vi "FeedbackDecode.vi"() -> ()   [LabVIEW 2020] (continued)
            n2136 = call "FeedbackDecode_MLComCtrl.vi"("DecodeClustIn"=w2282, "Mode"=T19."SendEvent") -> ()  [unwired: 6 in, 4 out]
          }
          event Value Change {
            n2137 = event-data() -> ()  [unwired: 1 in, 6 out]
            n2138 = local read "EncodeClust"() -> (w2298:T9)
            n2139 = call "FeedbackDecode_AdjParamsTable.vi"("StimClustIn"=w2298, "Mode"=enum16{"Set", "Add", "Sub"}."Add") -> ("StimClustOut"=w2296:T9)  [unwired: 1 in]
            n2140 = Bundle By Name(cluster=w2296, "AdjClust.Add"=FALSE ("AdjClust.Set")) -> (w2294:T9)
            n2141 = local read "LoopCnt"() -> (w2308:u64)
            n2142 = call "FeedbackDecode_Params2Preset.vi"("StimClustIn"=w2294) -> ("StimClustOut"=w2299:T9)  [unwired: 2 in]
            n2143 = Format Into String(w2308) -> (resulting string=w2300:string)  [unwired: 3 in, 1 out]
            n2144 = local read "NIPTime"() -> (w2304:dbl)
            n2145 = call "FeedbackDecode_BuildStimCmd.vi"("EncodeClustIn"=w2299) -> ("EncodeClustOut"=w2314:T9, "StimCmd"=w2293:string)  [unwired: 1 in]
            n2146 = local read "EventParamsFID"() -> (w2312:refnum<file>)
            n2147 = Concatenate Strings("UpdateStim:SS.EventID=" ("string"), w2300) -> (w2307:string)
            n2148 = call-poly "FeedbackDecode_VariablesToString.vi"("Format"="%0.0f", "ValueIn"=w2304, "FieldName"="NIPTime" ("Key Word")) -> ("StringOut"=w2301:string)  [unwired: 4 in]
            n2149 = local read "DecodeClust"() -> (w2313:T5)
            n2150 = Concatenate Strings(w2307, ";", w2293, w2301) -> (w2306:string)
            n2151 = call "FeedbackDecode_WriteTextEOL.vi"("text"=w2306, "refnum in"=w2312) -> ()  [unwired: 8 in, 2 out]
            n2152 = Bundle By Name(cluster=w2313, "EventStr"=w2306) -> (w2305:T5)
            n2153 = local write "StimCmd"(w2293) -> ()
            n2154 = local write "EncodeClust"(w2314) -> ()
            n2155 = call "FeedbackDecode_MLComCtrl.vi"("DecodeClustIn"=w2305, "Mode"=T19."SendEvent") -> ()  [unwired: 6 in, 4 out]
          }
          event Value Change {
            n2156 = event-data() -> ()  [unwired: 1 in, 6 out]
            n2157 = local read "EncodeClust"() -> (w2321:T9)
            n2158 = call "FeedbackDecode_AdjParamsTable.vi"("StimClustIn"=w2321, "Mode"=enum16{"Set", "Add", "Sub"}."Sub") -> ("StimClustOut"=w2319:T9)  [unwired: 1 in]
            n2159 = Bundle By Name(cluster=w2319, "AdjClust.Sub"=FALSE ("AdjClust.Set")) -> (w2317:T9)
            n2160 = local read "LoopCnt"() -> (w2331:u64)
            n2161 = call "FeedbackDecode_Params2Preset.vi"("StimClustIn"=w2317) -> ("StimClustOut"=w2322:T9)  [unwired: 2 in]
            n2162 = Format Into String(w2331) -> (resulting string=w2323:string)  [unwired: 3 in, 1 out]
            n2163 = local read "NIPTime"() -> (w2327:dbl)
            n2164 = call "FeedbackDecode_BuildStimCmd.vi"("EncodeClustIn"=w2322) -> ("EncodeClustOut"=w2337:T9, "StimCmd"=w2316:string)  [unwired: 1 in]
            n2165 = local read "EventParamsFID"() -> (w2335:refnum<file>)
            n2166 = Concatenate Strings("UpdateStim:SS.EventID=" ("string"), w2323) -> (w2330:string)
            n2167 = call-poly "FeedbackDecode_VariablesToString.vi"("Format"="%0.0f", "ValueIn"=w2327, "FieldName"="NIPTime" ("Key Word")) -> ("StringOut"=w2324:string)  [unwired: 4 in]
            n2168 = local read "DecodeClust"() -> (w2336:T5)
            n2169 = Concatenate Strings(w2330, ";", w2316, w2324) -> (w2329:string)
            n2170 = call "FeedbackDecode_WriteTextEOL.vi"("text"=w2329, "refnum in"=w2335) -> ()  [unwired: 8 in, 2 out]
            n2171 = Bundle By Name(cluster=w2336, "EventStr"=w2329) -> (w2328:T5)
            n2172 = local write "StimCmd"(w2316) -> ()
            n2173 = local write "EncodeClust"(w2337) -> ()
            n2174 = call "FeedbackDecode_MLComCtrl.vi"("DecodeClustIn"=w2328, "Mode"=T19."SendEvent") -> ()  [unwired: 6 in, 4 out]
          }
          event Value Change {
            n2175 = event-data() -> ()  [unwired: 1 in, 6 out]
            n2176 = local read "EncodeClust"() -> (w2351:T9)
            n2177 = Unbundle By Name(w2351) -> ("Sel"=w2344:bool[], "ParamsTable"=w2345:string[][], "SelPreset"=w2349:bool[])
            n2178 = while {
              shift-right: [w2377] -> w2343
              shift-left: w2344 -> [w2376]
              shift-right: [w2372] -> w2342
              shift-left: w2345 -> [w2373]
              stop <- w2370 stop-if-true
              n2179 = Search 1D Array(1D array=w2376, element=TRUE) -> (index of element=w2371:i32)  [unwired: 1 in]
              n2180 = Less Than 0?(x=w2371) -> (x < 0?=w2370:bool)
              n2181 = Delete From Array(array=w2376, length=1, index=w2371) -> (array with subset deleted=w2377:bool[])  [unwired: 1 out]
              n2182 = Delete From Array(array=w2373, length=1, index (row)=w2371) -> (array with subset deleted=w2372:string[][])  [unwired: 1 in, 1 out]
            }
            n2183 = Array Size(array=w2349) -> (size(s)=w2347:i32)
            n2184 = Initialize Array(FALSE, w2347) -> (w2350:bool[])
            n2185 = Bundle By Name(cluster=w2351, "Sel"=w2343, "ParamsTable"=w2342, "AdjClust.DeleteSel"=FALSE, "SelPreset"=w2350) -> (w2341:T9)
            n2186 = local read "LoopCnt"() -> (w2361:u64)
            n2187 = call "FeedbackDecode_UpdateParamsTable.vi"("StimClustIn"=w2341) -> ("StimClustOut"=w2340:T9)  [unwired: 2 in]
            n2188 = call "FeedbackDecode_Params2UEA.vi"("StimClustIn"=w2340) -> ("StimClustOut"=w2352:T9)  [unwired: 2 in]
            n2189 = Format Into String(w2361) -> (resulting string=w2353:string)  [unwired: 3 in, 1 out]
            n2190 = local read "NIPTime"() -> (w2357:dbl)
            n2191 = call "FeedbackDecode_BuildStimCmd.vi"("EncodeClustIn"=w2352) -> ("EncodeClustOut"=w2367:T9, "StimCmd"=w2339:string)  [unwired: 1 in]
            n2192 = local read "EventParamsFID"() -> (w2365:refnum<file>)
            n2193 = Concatenate Strings("DelStimParam:SS.EventID=" ("string"), w2353) -> (w2360:string)
            n2194 = call-poly "FeedbackDecode_VariablesToString.vi"("Format"="%0.0f", "ValueIn"=w2357, "FieldName"="NIPTime" ("Key Word")) -> ("StringOut"=w2354:string)  [unwired: 4 in]
            n2195 = local read "DecodeClust"() -> (w2366:T5)
            n2196 = Concatenate Strings(w2360, ";", w2339, w2354) -> (w2359:string)
            n2197 = call "FeedbackDecode_WriteTextEOL.vi"("text"=w2359, "refnum in"=w2365) -> ()  [unwired: 8 in, 2 out]
            n2198 = Bundle By Name(cluster=w2366, "EventStr"=w2359) -> (w2358:T5)
            n2199 = local write "StimCmd"(w2339) -> ()
            n2200 = local write "EncodeClust"(w2367) -> ()
            n2201 = call "FeedbackDecode_MLComCtrl.vi"("DecodeClustIn"=w2358, "Mode"=T19."SendEvent") -> ()  [unwired: 6 in, 4 out]
          }
          event Value Change {
            n2202 = event-data() -> ()  [unwired: 1 in, 6 out]
            n2203 = local read "EncodeClust"() -> (w2391:T9)
            n2204 = Unbundle By Name(w2391) -> ("SelPreset"=w2384:bool[], "PresetTable"=w2385:string[][], "Sel"=w2389:bool[])
            n2205 = while {
              shift-right: [w2417] -> w2383
              shift-left: w2384 -> [w2416]
              shift-right: [w2412] -> w2382
              shift-left: w2385 -> [w2413]
              stop <- w2410 stop-if-true
              n2206 = Search 1D Array(1D array=w2416, element=TRUE) -> (index of element=w2411:i32)  [unwired: 1 in]
              n2207 = Less Than 0?(x=w2411) -> (x < 0?=w2410:bool)
              n2208 = Delete From Array(array=w2416, length=1, index=w2411) -> (array with subset deleted=w2417:bool[])  [unwired: 1 out]
              n2209 = Delete From Array(array=w2413, length=1, index (row)=w2411) -> (array with subset deleted=w2412:string[][])  [unwired: 1 in, 1 out]
            }
            n2210 = Array Size(array=w2389) -> (size(s)=w2387:i32)
            n2211 = Initialize Array(FALSE, w2387) -> (w2390:bool[])
            n2212 = Bundle By Name(cluster=w2391, "SelPreset"=w2383, "PresetTable"=w2382, "PresetClust.Del"=FALSE ("AdjClust.DeleteSel"), "Sel"=w2390) -> (w2379:T9)
            n2213 = call "FeedbackDecode_UpdatePresetsTable.vi"("StimClustIn"=w2379) -> ("StimClustOut"=w2378:T9)  [unwired: 2 in]
            n2214 = local read "LoopCnt"() -> (w2401:u64)
            n2215 = call "FeedbackDecode_UpdateParamsTable.vi"("StimClustIn"=w2378) -> ("StimClustOut"=w2381:T9)  [unwired: 2 in]
            n2216 = call "FeedbackDecode_Params2UEA.vi"("StimClustIn"=w2381) -> ("StimClustOut"=w2392:T9)  [unwired: 2 in]
            n2217 = Format Into String(w2401) -> (resulting string=w2393:string)  [unwired: 3 in, 1 out]
            n2218 = local read "NIPTime"() -> (w2397:dbl)
            n2219 = call "FeedbackDecode_BuildStimCmd.vi"("EncodeClustIn"=w2392) -> ("EncodeClustOut"=w2407:T9, "StimCmd"=w2380:string)  [unwired: 1 in]
            n2220 = local read "EventParamsFID"() -> (w2405:refnum<file>)
            n2221 = Concatenate Strings("DelPreset:SS.EventID=" ("string"), w2393) -> (w2400:string)
            n2222 = call-poly "FeedbackDecode_VariablesToString.vi"("Format"="%0.0f", "ValueIn"=w2397, "FieldName"="NIPTime" ("Key Word")) -> ("StringOut"=w2394:string)  [unwired: 4 in]
            n2223 = local read "DecodeClust"() -> (w2406:T5)
            n2224 = Concatenate Strings(w2400, ";", w2380, w2394) -> (w2399:string)
            n2225 = call "FeedbackDecode_WriteTextEOL.vi"("text"=w2399, "refnum in"=w2405) -> ()  [unwired: 8 in, 2 out]
            n2226 = Bundle By Name(cluster=w2406, "EventStr"=w2399) -> (w2398:T5)
            n2227 = local write "StimCmd"(w2380) -> ()
            n2228 = local write "EncodeClust"(w2407) -> ()
            n2229 = call "FeedbackDecode_MLComCtrl.vi"("DecodeClustIn"=w2398, "Mode"=T19."SendEvent") -> ()  [unwired: 6 in, 4 out]
          }
          event Value Change {
            n2230 = event-data() -> ()  [unwired: 1 in, 6 out]
            n2231 = local read "EncodeClust"() -> (w2428:T9)
            n2232 = Unbundle By Name(w2428) -> ("SelPreset"=w2424:bool[])
            n2233 = Array Size(array=w2424) -> (size(s)=w2426:i32)
            n2234 = Initialize Array(FALSE, w2426) -> (w2427:bool[])
            n2235 = Bundle By Name(cluster=w2428, "ParamsTable"=string[][] [], "Sel"=bool[] [], "UEAArray"=T25 [{"Boolean 1"=FALSE, "Boolean 2"=FALSE, "Boolean 3"=FALSE, "Boolean 4"=FALSE, "Boolean 5"=FALSE, "Boolean 6"=FALSE, "Boolean 7"=FALSE, "Boolean 8"=FALSE, "Boolean 9"=FALSE, "Boolean 10"=FALSE, "Boolean 11"=FALSE, "Boolean 12"=FALSE, "Boolean 13"=FALSE, "Boolean 14"=FALSE, "Boolean 15"=FALSE, "Boolean 16"=FALSE, "Boolean 17"=FALSE, "Boolean 18"=FALSE, "Boolean 19"=FALSE, "Boolean 20"=FALSE, "Boolean 21"=FALSE, "Boolean 22"=FALSE, "Boolean 23"=FALSE, "Boolean 24"=FALSE, "Boolean 25"=FALSE, "Boolean 26"=FALSE, "Boolean 27"=FALSE, "Boolean 28"=FALSE, "Boolean 29"=FALSE, "Boolean 30"=FALSE, "Boolean 31"=FALSE, "Boolean 32"=FALSE, "Boolean 33"=FALSE, "Boolean 34"=FALSE, "Boolean 35"=FALSE, "Boolean 36"=FALSE, "Boolean 37"=FALSE, "Boolean 38"=FALSE, "Boolean 39"=FALSE, "Boolean 40"=FALSE, "Boolean 41"=FALSE, "Boolean 42"=FALSE, "Boolean 43"=FALSE, "Boolean 44"=FALSE, "Boolean 45"=FALSE, "Boolean 46"=FALSE, "Boolean 47"=FALSE, "Boolean 48"=FALSE, "Boolean 49"=FALSE, "Boolean 50"=FALSE, "Boolean 51"=FALSE, "Boolean 52"=FALSE, "Boolean 53"=FALSE, "Boolean 54"=FALSE, "Boolean 55"=FALSE, "Boolean 56"=FALSE, "Boolean 57"=FALSE, "Boolean 58"=FALSE, "Boolean 59"=FALSE, "Boolean 60"=FALSE, "Boolean 61"=FALSE, "Boolean 62"=FALSE, "Boolean 63"=FALSE, "Boolean 64"=FALSE, "Boolean 65"=FALSE, "Boolean 66"=FALSE, "Boolean 67"=FALSE, "Boolean 68"=FALSE, "Boolean 69"=FALSE, "Boolean 70"=FALSE, "Boolean 71"=FALSE, "Boolean 72"=FALSE, "Boolean 73"=FALSE, "Boolean 74"=FALSE, "Boolean 75"=FALSE, "Boolean 76"=FALSE, "Boolean 77"=FALSE, "Boolean 78"=FALSE, "Boolean 79"=FALSE, "Boolean 80"=FALSE, "Boolean 81"=FALSE, "Boolean 82"=FALSE, "Boolean 83"=FALSE, "Boolean 84"=FALSE, "Boolean 85"=FALSE, "Boolean 86"=FALSE, "Boolean 87"=FALSE, "Boolean 88"=FALSE, "Boolean 89"=FALSE, "Boolean 90"=FALSE, "Boolean 91"=FALSE, "Boolean 92"=FALSE, "Boolean 93"=FALSE, "Boolean 94"=FALSE, "Boolean 95"=FALSE, "Boolean 96"=FALSE, "Boolean 97"=FALSE, "Boolean 98"=FALSE, "Boolean 99"=FALSE, "Boolean 100"=FALSE}, {"Boolean 1"=FALSE, "Boolean 2"=FALSE, "Boolean 3"=FALSE, "Boolean 4"=FALSE, "Boolean 5"=FALSE, "Boolean 6"=FALSE, "Boolean 7"=FALSE, "Boolean 8"=FALSE, "Boolean 9"=FALSE, "Boolean 10"=FALSE, "Boolean 11"=FALSE, "Boolean 12"=FALSE, "Boolean 13"=FALSE, "Boolean 14"=FALSE, "Boolean 15"=FALSE, "Boolean 16"=FALSE, "Boolean 17"=FALSE, "Boolean 18"=FALSE, "Boolean 19"=FALSE, "Boolean 20"=FALSE, "Boolean 21"=FALSE, "Boolean 22"=FALSE, "Boolean 23"=FALSE, "Boolean 24"=FALSE, "Boolean 25"=FALSE, "Boolean 26"=FALSE, "Boolean 27"=FALSE, "Boolean 28"=FALSE, "Boolean 29"=FALSE, "Boolean 30"=FALSE, "Boolean 31"=FALSE, "Boolean 32"=FALSE, "Boolean 33"=FALSE, "Boolean 34"=FALSE, "Boolean 35"=FALSE, "Boolean 36"=FALSE, "Boolean 37"=FALSE, "Boolean 38"=FALSE, "Boolean 39"=FALSE, "Boolean 40"=FALSE, "Boolean 41"=FALSE, "Boolean 42"=FALSE, "Boolean 43"=FALSE, "Boolean 44"=FALSE, "Boolean 45"=FALSE, "Boolean 46"=FALSE, "Boolean 47"=FALSE, "Boolean 48"=FALSE, "Boolean 49"=FALSE, "Boolean 50"=FALSE, "Boolean 51"=FALSE, "Boolean 52"=FALSE, "Boolean 53"=FALSE, "Boolean 54"=FALSE, "Boolean 55"=FALSE, "Boolean 56"=FALSE, "Boolean 57"=FALSE, "Boolean 58"=FALSE, "Boolean 59"=FALSE, "Boolean 60"=FALSE, "Boolean 61"=FALSE, "Boolean 62"=FALSE, "Boolean 63"=FALSE, "Boolean 64"=FALSE, "Boolean 65"=FALSE, "Boolean 66"=FALSE, "Boolean 67"=FALSE, "Boolean 68"=FALSE, "Boolean 69"=FALSE, "Boolean 70"=FALSE, "Boolean 71"=FALSE, "Boolean 72"=FALSE, "Boolean 73"=FALSE, "Boolean 74"=FALSE, "Boolean 75"=FALSE, "Boolean 76"=FALSE, "Boolean 77"=FALSE, "Boolean 78"=FALSE, "Boolean 79"=FALSE, "Boolean 80"=FALSE, "Boolean 81"=FALSE, "Boolean 82"=FALSE, "Boolean 83"=FALSE, "Boolean 84"=FALSE, "Boolean 85"=FALSE, "Boolean 86"=FALSE, "Boolean 87"=FALSE, "Boolean 88"=FALSE, "Boolean 89"=FALSE, "Boolean 90"=FALSE, "Boolean 91"=FALSE, "Boolean 92"=FALSE, "Boolean 93"=FALSE, "Boolean 94"=FALSE, "Boolean 95"=FALSE, "Boolean 96"=FALSE, "Boolean 97"=FALSE, "Boolean 98"=FALSE, "Boolean 99"=FALSE, "Boolean 100"=FALSE}], "AdjClust.ClearTable"=FALSE, "SelPreset"=w2427) -> (w2419:T9)
            n2236 = local read "LoopCnt"() -> (w2439:u64)
            n2237 = call "FeedbackDecode_UpdateParamsTable.vi"("StimClustIn"=w2419) -> ("StimClustOut"=w2429:T9)  [unwired: 2 in]
            n2238 = call "FeedbackDecode_Params2UEA.vi"("StimClustIn"=w2429) -> ("StimClustOut"=w2430:T9)  [unwired: 2 in]
            n2239 = Format Into String(w2439) -> (resulting string=w2431:string)  [unwired: 3 in, 1 out]
            n2240 = local read "NIPTime"() -> (w2435:dbl)
            n2241 = call "FeedbackDecode_BuildStimCmd.vi"("EncodeClustIn"=w2430) -> ("EncodeClustOut"=w2445:T9, "StimCmd"=w2418:string)  [unwired: 1 in]
            n2242 = local read "EventParamsFID"() -> (w2443:refnum<file>)
            n2243 = Concatenate Strings("ClearStimParams:SS.EventID=" ("string"), w2431) -> (w2438:string)
            n2244 = call-poly "FeedbackDecode_VariablesToString.vi"("Format"="%0.0f", "ValueIn"=w2435, "FieldName"="NIPTime" ("Key Word")) -> ("StringOut"=w2432:string)  [unwired: 4 in]
            n2245 = local read "DecodeClust"() -> (w2444:T5)
            n2246 = Concatenate Strings(w2438, ";", w2418, w2432) -> (w2437:string)
            n2247 = call "FeedbackDecode_WriteTextEOL.vi"("text"=w2437, "refnum in"=w2443) -> ()  [unwired: 8 in, 2 out]
            n2248 = Bundle By Name(cluster=w2444, "EventStr"=w2437) -> (w2436:T5)
            n2249 = local write "StimCmd"(w2418) -> ()
            n2250 = local write "EncodeClust"(w2445) -> ()
            n2251 = call "FeedbackDecode_MLComCtrl.vi"("DecodeClustIn"=w2436, "Mode"=T19."SendEvent") -> ()  [unwired: 6 in, 4 out]
          }
          event Value Change {
            n2252 = event-data() -> ()  [unwired: 1 in, 6 out]
            n2253 = local read "EncodeClust"() -> (w2458:T9)
            n2254 = Unbundle By Name(w2458) -> ("Sel"=w2454:bool[])
            n2255 = Array Size(array=w2454) -> (size(s)=w2456:i32)
            n2256 = Initialize Array(FALSE, w2456) -> (w2457:bool[])
            n2257 = Bundle By Name(cluster=w2458, "PresetTable"=string[][] [] ("ParamsTable"), "SelPreset"=bool[] [] ("Sel"), "UEAArray"=T25 [{"Boolean 1"=FALSE, "Boolean 2"=FALSE, "Boolean 3"=FALSE, "Boolean 4"=FALSE, "Boolean 5"=FALSE, "Boolean 6"=FALSE, "Boolean 7"=FALSE, "Boolean 8"=FALSE, "Boolean 9"=FALSE, "Boolean 10"=FALSE, "Boolean 11"=FALSE, "Boolean 12"=FALSE, "Boolean 13"=FALSE, "Boolean 14"=FALSE, "Boolean 15"=FALSE, "Boolean 16"=FALSE, "Boolean 17"=FALSE, "Boolean 18"=FALSE, "Boolean 19"=FALSE, "Boolean 20"=FALSE, "Boolean 21"=FALSE, "Boolean 22"=FALSE, "Boolean 23"=FALSE, "Boolean 24"=FALSE, "Boolean 25"=FALSE, "Boolean 26"=FALSE, "Boolean 27"=FALSE, "Boolean 28"=FALSE, "Boolean 29"=FALSE, "Boolean 30"=FALSE, "Boolean 31"=FALSE, "Boolean 32"=FALSE, "Boolean 33"=FALSE, "Boolean 34"=FALSE, "Boolean 35"=FALSE, "Boolean 36"=FALSE, "Boolean 37"=FALSE, "Boolean 38"=FALSE, "Boolean 39"=FALSE, "Boolean 40"=FALSE, "Boolean 41"=FALSE, "Boolean 42"=FALSE, "Boolean 43"=FALSE, "Boolean 44"=FALSE, "Boolean 45"=FALSE, "Boolean 46"=FALSE, "Boolean 47"=FALSE, "Boolean 48"=FALSE, "Boolean 49"=FALSE, "Boolean 50"=FALSE, "Boolean 51"=FALSE, "Boolean 52"=FALSE, "Boolean 53"=FALSE, "Boolean 54"=FALSE, "Boolean 55"=FALSE, "Boolean 56"=FALSE, "Boolean 57"=FALSE, "Boolean 58"=FALSE, "Boolean 59"=FALSE, "Boolean 60"=FALSE, "Boolean 61"=FALSE, "Boolean 62"=FALSE, "Boolean 63"=FALSE, "Boolean 64"=FALSE, "Boolean 65"=FALSE, "Boolean 66"=FALSE, "Boolean 67"=FALSE, "Boolean 68"=FALSE, "Boolean 69"=FALSE, "Boolean 70"=FALSE, "Boolean 71"=FALSE, "Boolean 72"=FALSE, "Boolean 73"=FALSE, "Boolean 74"=FALSE, "Boolean 75"=FALSE, "Boolean 76"=FALSE, "Boolean 77"=FALSE, "Boolean 78"=FALSE, "Boolean 79"=FALSE, "Boolean 80"=FALSE, "Boolean 81"=FALSE, "Boolean 82"=FALSE, "Boolean 83"=FALSE, "Boolean 84"=FALSE, "Boolean 85"=FALSE, "Boolean 86"=FALSE, "Boolean 87"=FALSE, "Boolean 88"=FALSE, "Boolean 89"=FALSE, "Boolean 90"=FALSE, "Boolean 91"=FALSE, "Boolean 92"=FALSE, "Boolean 93"=FALSE, "Boolean 94"=FALSE, "Boolean 95"=FALSE, "Boolean 96"=FALSE, "Boolean 97"=FALSE, "Boolean 98"=FALSE, "Boolean 99"=FALSE, "Boolean 100"=FALSE}, {"Boolean 1"=FALSE, "Boolean 2"=FALSE, "Boolean 3"=FALSE, "Boolean 4"=FALSE, "Boolean 5"=FALSE, "Boolean 6"=FALSE, "Boolean 7"=FALSE, "Boolean 8"=FALSE, "Boolean 9"=FALSE, "Boolean 10"=FALSE, "Boolean 11"=FALSE, "Boolean 12"=FALSE, "Boolean 13"=FALSE, "Boolean 14"=FALSE, "Boolean 15"=FALSE, "Boolean 16"=FALSE, "Boolean 17"=FALSE, "Boolean 18"=FALSE, "Boolean 19"=FALSE, "Boolean 20"=FALSE, "Boolean 21"=FALSE, "Boolean 22"=FALSE, "Boolean 23"=FALSE, "Boolean 24"=FALSE, "Boolean 25"=FALSE, "Boolean 26"=FALSE, "Boolean 27"=FALSE, "Boolean 28"=FALSE, "Boolean 29"=FALSE, "Boolean 30"=FALSE, "Boolean 31"=FALSE, "Boolean 32"=FALSE, "Boolean 33"=FALSE, "Boolean 34"=FALSE, "Boolean 35"=FALSE, "Boolean 36"=FALSE, "Boolean 37"=FALSE, "Boolean 38"=FALSE, "Boolean 39"=FALSE, "Boolean 40"=FALSE, "Boolean 41"=FALSE, "Boolean 42"=FALSE, "Boolean 43"=FALSE, "Boolean 44"=FALSE, "Boolean 45"=FALSE, "Boolean 46"=FALSE, "Boolean 47"=FALSE, "Boolean 48"=FALSE, "Boolean 49"=FALSE, "Boolean 50"=FALSE, "Boolean 51"=FALSE, "Boolean 52"=FALSE, "Boolean 53"=FALSE, "Boolean 54"=FALSE, "Boolean 55"=FALSE, "Boolean 56"=FALSE, "Boolean 57"=FALSE, "Boolean 58"=FALSE, "Boolean 59"=FALSE, "Boolean 60"=FALSE, "Boolean 61"=FALSE, "Boolean 62"=FALSE, "Boolean 63"=FALSE, "Boolean 64"=FALSE, "Boolean 65"=FALSE, "Boolean 66"=FALSE, "Boolean 67"=FALSE, "Boolean 68"=FALSE, "Boolean 69"=FALSE, "Boolean 70"=FALSE, "Boolean 71"=FALSE, "Boolean 72"=FALSE, "Boolean 73"=FALSE, "Boolean 74"=FALSE, "Boolean 75"=FALSE, "Boolean 76"=FALSE, "Boolean 77"=FALSE, "Boolean 78"=FALSE, "Boolean 79"=FALSE, "Boolean 80"=FALSE, "Boolean 81"=FALSE, "Boolean 82"=FALSE, "Boolean 83"=FALSE, "Boolean 84"=FALSE, "Boolean 85"=FALSE, "Boolean 86"=FALSE, "Boolean 87"=FALSE, "Boolean 88"=FALSE, "Boolean 89"=FALSE, "Boolean 90"=FALSE, "Boolean 91"=FALSE, "Boolean 92"=FALSE, "Boolean 93"=FALSE, "Boolean 94"=FALSE, "Boolean 95"=FALSE, "Boolean 96"=FALSE, "Boolean 97"=FALSE, "Boolean 98"=FALSE, "Boolean 99"=FALSE, "Boolean 100"=FALSE}], "PresetClust.Clear"=FALSE ("AdjClust.ClearTable"), "Sel"=w2457) -> (w2448:T9)
            n2258 = call "FeedbackDecode_UpdatePresetsTable.vi"("StimClustIn"=w2448) -> ("StimClustOut"=w2447:T9)  [unwired: 2 in]
            n2259 = local read "LoopCnt"() -> (w2469:u64)
            n2260 = call "FeedbackDecode_UpdateParamsTable.vi"("StimClustIn"=w2447) -> ("StimClustOut"=w2459:T9)  [unwired: 2 in]
            n2261 = call "FeedbackDecode_Params2UEA.vi"("StimClustIn"=w2459) -> ("StimClustOut"=w2460:T9)  [unwired: 2 in]
            n2262 = Format Into String(w2469) -> (resulting string=w2461:string)  [unwired: 3 in, 1 out]
            n2263 = local read "NIPTime"() -> (w2465:dbl)
            n2264 = call "FeedbackDecode_BuildStimCmd.vi"("EncodeClustIn"=w2460) -> ("EncodeClustOut"=w2475:T9, "StimCmd"=w2449:string)  [unwired: 1 in]
            n2265 = local read "EventParamsFID"() -> (w2473:refnum<file>)
            n2266 = Concatenate Strings("ClearPresets:SS.EventID=" ("string"), w2461) -> (w2468:string)
            n2267 = call-poly "FeedbackDecode_VariablesToString.vi"("Format"="%0.0f", "ValueIn"=w2465, "FieldName"="NIPTime" ("Key Word")) -> ("StringOut"=w2462:string)  [unwired: 4 in]
            n2268 = local read "DecodeClust"() -> (w2474:T5)
            n2269 = Concatenate Strings(w2468, ";", w2449, w2462) -> (w2467:string)
            n2270 = call "FeedbackDecode_WriteTextEOL.vi"("text"=w2467, "refnum in"=w2473) -> ()  [unwired: 8 in, 2 out]
            n2271 = Bundle By Name(cluster=w2474, "EventStr"=w2467) -> (w2466:T5)
            n2272 = local write "StimCmd"(w2449) -> ()
            n2273 = local write "EncodeClust"(w2475) -> ()
            n2274 = call "FeedbackDecode_MLComCtrl.vi"("DecodeClustIn"=w2466, "Mode"=T19."SendEvent") -> ()  [unwired: 6 in, 4 out]
          }
          event Value Change {
            n2275 = event-data() -> ()  [unwired: 1 in, 6 out]
            n2276 = local read "EncodeClust"() -> (w2485:T9)
            n2277 = Bundle By Name(cluster=w2485, "Stim"=FALSE) -> (w2483:T9)
            n2278 = call "FeedbackDecode_BuildStimCmd.vi"("EncodeClustIn"=w2483) -> ("EncodeClustOut"=w2495:T9, "StimCmd"=w2477:string)  [unwired: 1 in]
            n2279 = local read "LoopCnt"() -> (w2489:u64)
            n2280 = local read "NIPTime"() -> (w2482:dbl)
            n2281 = local write "EncodeClust"(w2495) -> ()
            n2282 = local write "StimCmd"(w2477) -> ()
            n2283 = Format Into String(w2489) -> (resulting string=w2478:string)  [unwired: 3 in, 1 out]
            n2284 = call-poly "FeedbackDecode_VariablesToString.vi"("Format"="%0.0f", "ValueIn"=w2482, "FieldName"="NIPTime" ("Key Word")) -> ("StringOut"=w2479:string)  [unwired: 4 in]
            n2285 = local read "EventParamsFID"() -> (w2493:refnum<file>)
            n2286 = Concatenate Strings("ChangeStimMode:SS.EventID=" ("string"), w2478) -> (w2488:string)
            n2287 = local read "DecodeClust"() -> (w2494:T5)
            n2288 = Concatenate Strings(w2488, ";", w2477, w2479) -> (w2487:string)
            n2289 = call "FeedbackDecode_WriteTextEOL.vi"("text"=w2487, "refnum in"=w2493) -> ()  [unwired: 8 in, 2 out]
            n2290 = Bundle By Name(cluster=w2494, "EventStr"=w2487) -> (w2486:T5)
            n2291 = call "FeedbackDecode_MLComCtrl.vi"("DecodeClustIn"=w2486, "Mode"=T19."SendEvent") -> ()  [unwired: 6 in, 4 out]
          }
          event Value Change {
            n2292 = event-data() -> ()  [unwired: 1 in, 6 out]
            n2293 = local read "EncodeClust"() -> (w2497:T9)
            n2294 = call "FeedbackDecode_BuildStimCmd.vi"("EncodeClustIn"=w2497) -> ("EncodeClustOut"=w2513:T9, "StimCmd"=w2498:string)  [unwired: 1 in]
            n2295 = local read "LoopCnt"() -> (w2507:u64)
            n2296 = local read "NIPTime"() -> (w2503:dbl)
            n2297 = local write "EncodeClust"(w2513) -> ()
            n2298 = local write "StimCmd"(w2498) -> ()
            n2299 = Format Into String(w2507) -> (resulting string=w2499:string)  [unwired: 3 in, 1 out]
            n2300 = call-poly "FeedbackDecode_VariablesToString.vi"("Format"="%0.0f", "ValueIn"=w2503, "FieldName"="NIPTime" ("Key Word")) -> ("StringOut"=w2500:string)  [unwired: 4 in]
            n2301 = local read "EventParamsFID"() -> (w2511:refnum<file>)
            n2302 = Concatenate Strings("ChangeManualType:SS.EventID=" ("string"), w2499) -> (w2506:string)
            n2303 = local read "DecodeClust"() -> (w2512:T5)
            n2304 = Concatenate Strings(w2506, ";", w2498, w2500) -> (w2505:string)
            n2305 = call "FeedbackDecode_WriteTextEOL.vi"("text"=w2505, "refnum in"=w2511) -> ()  [unwired: 8 in, 2 out]
            n2306 = Bundle By Name(cluster=w2512, "EventStr"=w2505) -> (w2504:T5)
            n2307 = call "FeedbackDecode_MLComCtrl.vi"("DecodeClustIn"=w2504, "Mode"=T19."SendEvent") -> ()  [unwired: 6 in, 4 out]
          }
          event Value Change {
            n2308 = event-data() -> ("NewVal"=w2515:bool)  [unwired: 1 in, 5 out]
            n2309 = case shown="True" w2515 {
              frame False {
                n2310 = local write "PulseStim"(FALSE ("PulseStim")) -> ()
                n2311 = local write "BaseCnt3"(-inf) -> ()
                n2312 = local read "EncodeClust"() -> (w2534:T9)
                n2313 = local read "LoopCnt"() -> (w2528:u64)
                n2314 = call "FeedbackDecode_BuildStimCmd.vi"("EncodeClustIn"=w2534) -> ("EncodeClustOut"=w2533:T9, "StimCmd"=w2517:string)  [unwired: 1 in]
                n2315 = local read "NIPTime"() -> (w2524:dbl)
                n2316 = Format Into String(w2528) -> (resulting string=w2520:string)  [unwired: 3 in, 1 out]
                n2317 = local write "EncodeClust"(w2533) -> ()
                n2318 = local read "EventParamsFID"() -> (w2531:refnum<file>)
                n2319 = Concatenate Strings("ManualStim:SS.EventID=" ("string"), w2520, ";" ("string")) -> (w2527:string)
                n2320 = call-poly "FeedbackDecode_VariablesToString.vi"("Format"="%0.0f", "ValueIn"=w2524, "FieldName"="NIPTime" ("Key Word")) -> ("StringOut"=w2521:string)  [unwired: 4 in]
                n2321 = local write "StimCmd"(w2517) -> ()
                n2322 = Concatenate Strings(w2527, "SS.PulseStim=0;" ("string"), w2517, w2521) -> (w2526:string)
                n2323 = local read "DecodeClust"() -> (w2532:T5)
                n2324 = call "FeedbackDecode_WriteTextEOL.vi"("text"=w2526, "refnum in"=w2531) -> ()  [unwired: 8 in, 2 out]
                n2325 = Bundle By Name(cluster=w2532, "EventStr"=w2526) -> (w2525:T5)
                n2326 = call "FeedbackDecode_MLComCtrl.vi"("DecodeClustIn"=w2525, "Mode"=T19."SendEvent") -> ()  [unwired: 6 in, 4 out]
              }
              frame True {
                n2327 = local read "EncodeClust"() -> (w2540:T9)
                n2328 = local write "PulseStim"(FALSE ("PulseStim")) -> ()
                n2329 = Unbundle By Name(w2540) -> ("Train Period"=w2541:dbl)
                n2330 = local read "EncodeClust"() -> (w2559:T9)
                n2331 = local read "LoopCnt"() -> (w2538:u64)
                n2332 = expression code="x*100"(w2541) -> (w2539:dbl)
                n2333 = local read "LoopCnt"() -> (w2553:u64)
                n2334 = Add(x=w2538, y=w2539) -> (x+y=w2537:dbl)
                n2335 = call "FeedbackDecode_BuildStimCmd.vi"("EncodeClustIn"=w2559) -> ("EncodeClustOut"=w2558:T9, "StimCmd"=w2542:string)  [unwired: 1 in]
                n2336 = local write "BaseCnt3"(w2537) -> ()
                n2337 = local read "NIPTime"() -> (w2549:dbl)
                n2338 = Format Into String(w2553) -> (resulting string=w2545:string)  [unwired: 3 in, 1 out]
                n2339 = local write "EncodeClust"(w2558) -> ()
                n2340 = Concatenate Strings("ManualStim:SS.EventID=" ("string"), w2545, ";" ("string")) -> (w2552:string)
                n2341 = call-poly "FeedbackDecode_VariablesToString.vi"("Format"="%0.0f", "ValueIn"=w2549, "FieldName"="NIPTime" ("Key Word")) -> ("StringOut"=w2546:string)  [unwired: 4 in]
                n2342 = local read "EventParamsFID"() -> (w2556:refnum<file>)
                n2343 = local write "StimCmd"(w2542) -> ()
                n2344 = Concatenate Strings(w2552, "SS.PulseStim=1;" ("string"), w2542, w2546) -> (w2551:string)
                n2345 = local read "DecodeClust"() -> (w2557:T5)
                n2346 = call "FeedbackDecode_WriteTextEOL.vi"("text"=w2551, "refnum in"=w2556) -> ()  [unwired: 8 in, 2 out]
                n2347 = Bundle By Name(cluster=w2557, "EventStr"=w2551) -> (w2550:T5)
                n2348 = call "FeedbackDecode_MLComCtrl.vi"("DecodeClustIn"=w2550, "Mode"=T19."SendEvent") -> ()  [unwired: 6 in, 4 out]
              }
            }
          }
          event Value Change {
            n2349 = event-data() -> ()  [unwired: 1 in, 6 out]
            n2350 = local read "EncodeClust"() -> (w2577:T9)
            n2351 = call "FeedbackDecode_BuildStimCmd.vi"("EncodeClustIn"=w2577) -> ("EncodeClustOut"=w2576:T9, "StimCmd"=w2561:string)  [unwired: 1 in]
            n2352 = local read "LoopCnt"() -> (w2571:u64)
            n2353 = local write "EncodeClust"(w2576) -> ()
            n2354 = local read "NIPTime"() -> (w2567:dbl)
            n2355 = Format Into String(w2571) -> (resulting string=w2562:string)  [unwired: 3 in, 1 out]
            n2356 = call-poly "FeedbackDecode_VariablesToString.vi"("Format"="%0.0f", "ValueIn"=w2567, "FieldName"="NIPTime" ("Key Word")) -> ("StringOut"=w2564:string)  [unwired: 4 in]
            n2357 = local read "EventParamsFID"() -> (w2574:refnum<file>)
            n2358 = Concatenate Strings("ChangeStimStep:SS.EventID=" ("string"), w2562) -> (w2570:string)
            n2359 = local write "StimCmd"(w2561) -> ()
            n2360 = local read "DecodeClust"() -> (w2575:T5)
            n2361 = Concatenate Strings(w2570, ";", w2561, w2564) -> (w2569:string)
            n2362 = call "FeedbackDecode_WriteTextEOL.vi"("text"=w2569, "refnum in"=w2574) -> ()  [unwired: 8 in, 2 out]
            n2363 = Bundle By Name(cluster=w2575, "EventStr"=w2569) -> (w2568:T5)
